vi "Keithley DMM7510 Continuous Acquisition.vi"() -> ()   [LabVIEW 2016]
doc: "This example shows how to configure a measurement, set up triggering, trigger a measurement, and retrieve a measurement. It shows how to use the low-level Data VIs to retrieve data from the DMM."
uses:
  Keithley DMM7510.lvlib
panel:
  in  "Function":u16(ring) items=["Voltage: DC", "Voltage: AC", "Current: DC", "Current: AC", "2W Resistance", "4W Resistance", "Diode", "Capacitance", "Temperature", "Continuity", "Frequency", "Period", "Ratio"]
  in  "Sample Count (10)":i32=10 format="%#.6g"
  in  "Timeout (10000 ms)":i32=10000 format="%#.6g"
  out "Waveform Chart":dbl[](graph)
  in  "VISA resource name":refnum<visa-resource-name>
  # "(c) 2015 Keithley Instruments,,  ALL RIGHTS RESERVED."
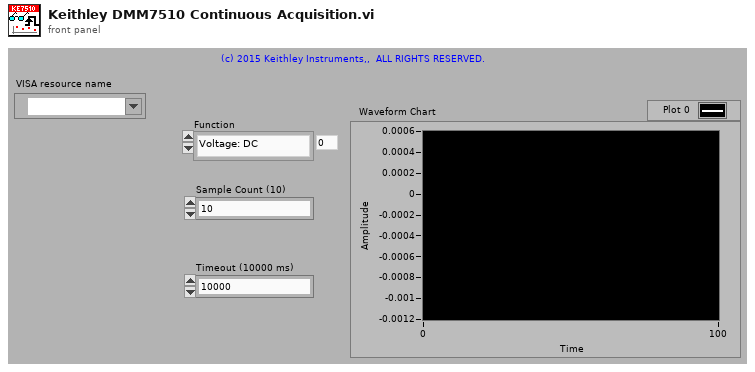
[diagram p1: front panel]
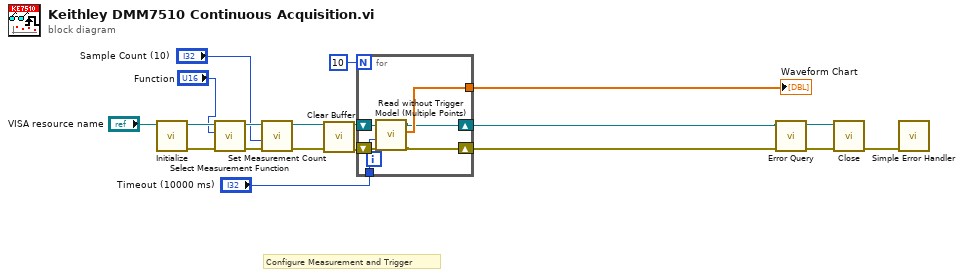
[diagram p0: block diagram]
diagram:
  # "Configure Measurement and Trigger"
  n1 = call "Initialize.vi"("VISA resource name"="VISA resource name") -> ("error out"=w15:errorcluster, "VISA resource name out"=w14:refnum<visa-resource-name>)  [unwired: 9 in]
  n2 = call "Select Measurement Function.vi"("error in (no error)"=w15, "Function"="Function", "VISA resource name"=w14) -> ("error out"=w12:errorcluster, "VISA resource name out"=w11:refnum<visa-resource-name>)  [unwired: 7 in]
  n3 = call "Set Measurement Count.vi"("error in (no error)"=w12, "Count"="Sample Count (10)", "VISA resource name"=w11) -> ("error out"=w5:errorcluster, "VISA resource name out"=w4:refnum<visa-resource-name>)  [unwired: 7 in]
  n4 = call "Clear Buffer.vi"("VISA resource name"=w4, "error in (no error)"=w5) -> ("VISA resource name out"=w3:refnum<visa-resource-name>, "error out"=w2:errorcluster)  [unwired: 12 in]
  n5 = for {
    N: 10 -> [_]
    tunnel: "Timeout (10000 ms)" -> [w25]
    tunnel: [w24] -> w8
    shift-right: [w23] -> w7
    shift-left: w3 -> [w21]
    shift-right: [w22] -> w6
    shift-left: w2 -> [w20]
    n6 = call "Read without Trigger Model (Multiple Points).vi"("error in (no error)"=w20, "Timeout (10000 ms)"=w25, "VISA resource name"=w21) -> ("error out"=w22:errorcluster, "Measurements"=w24:dbl[], "VISA resource name out"=w23:refnum<visa-resource-name>)  [unwired: 5 in, 1 out]
  }
  "Waveform Chart" <- w8
  n7 = call "Error Query.vi"("error in (no error)"=w6, "VISA resource name"=w7) -> ("error out"=w16:errorcluster, "VISA resource name out"=w17:refnum<visa-resource-name>)  [unwired: 6 in, 2 out]
  n8 = call "Close.vi"("error in (no error)"=w16, "VISA resource name"=w17) -> ("error out"=w18:errorcluster)  [unwired: 9 in]
  n9 = call <vilib>:"Simple Error Handler.vi"("error in (no error)"=w18) -> ()  [unwired: 4 in, 5 out]
